vi "GetConditions.vi"(6 "condition type":T3, 7 "data group":string, 8 "error in (no error)":errorcluster, 9 "operating state":i32, 11 "operating states in":variant) -> (0 "error out":errorcluster, 1 "expression":string, 2 "conditions":T1[](array[typedef]), 3 "operating states out":variant, 4 "weight":i32)   [LabVIEW 2017, in "OpState.lvlib"]
uses:
  <vilib>/addons/InsightCM/Devices/Shared/Common/OpState/OpState.lvlib
  <vilib>/addons/InsightCM/Devices/Shared/Common/OpState/controls/ConditionType.ctl
  <vilib>/addons/InsightCM/Devices/Shared/Common/Trigger/controls/TriggerCondition.ctl
  <vilib>/addons/InsightCM/MessageBus/Base/controls/Condition.ctl
  <vilib>/addons/InsightCM/Devices/Shared/Common/OpState/controls/TriggerOperatingState.ctl
  <vilib>/addons/InsightCM/MessageBus/Base/controls/KeyValuePair.ctl
  <vilib>/addons/InsightCM/Devices/Shared/Common/Trigger/Trigger.lvlib
  <vilib>/addons/InsightCM/Utilities/PropertyHelpers/PropertyHelpers.lvlib
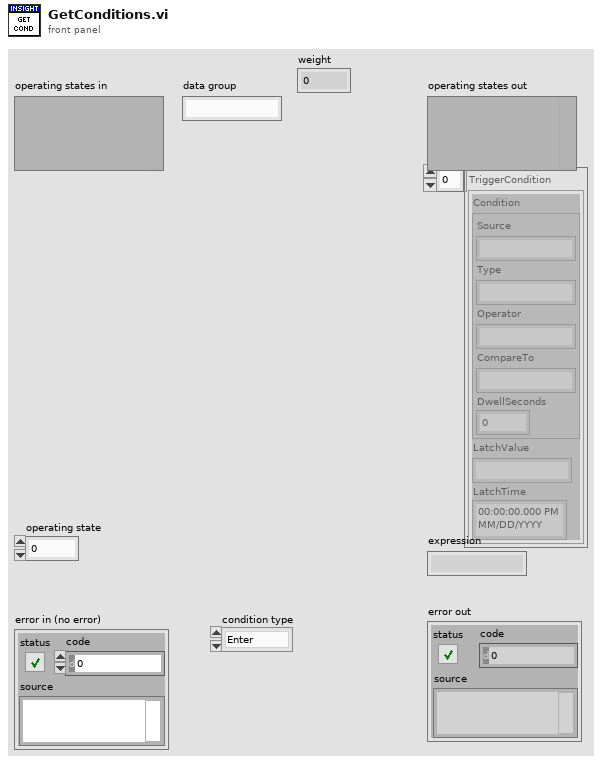
[diagram p1: front panel]
types:
  T1 = typedef "Trigger.lvlib/TriggerCondition.ctl" = cluster{"Condition":T2, "LatchValue":string, "LatchTime":timestamp}
  T2 = typedef "Condition.ctl" = cluster{"Source":string, "Type":string, "Operator":string, "CompareTo":string, "DwellSeconds":dbl}
  T3 = typedef "OpState.lvlib/ConditionType.ctl" = enum16{"Enter", "Exit"}
  T4 = typedef "OpState.lvlib/TriggerOperatingState.ctl" = cluster{"Id":string, "Name":string, "Properties":T5[], "EnterExpression":string, "EnterConditions":T1[], "ExitExpression":string, "ExitConditions":T1[]}
  T5 = typedef "KeyValuePair.ctl" = cluster{"Key":string, "Value":string}
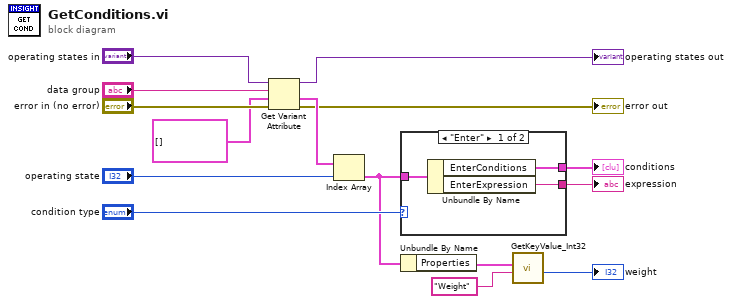
[diagram p0: block diagram]
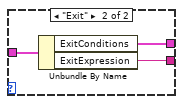
[diagram p2: hidden frame]
diagram:
  n1 = Get Variant Attribute(Variant="operating states in", name="data group", default value (empty Variant)=T4[] [] ("OperatingStates"), error in="error in (no error)") -> (duplicate Variant=→"operating states out":variant, value=w11:T4[], error out=→"error out":errorcluster)  [unwired: 1 out]
  n2 = Index Array(array=w11, index="operating state") -> (element=w4:T4)
  n3 = case shown="\"Enter\"" "condition type" {
    tunnel: w4 -> [w18 w21]
    tunnel: [w17 w20] -> w7
    tunnel: [w16 w19] -> w6
    frame "Enter" {
      n4 = Unbundle By Name(w18) -> ("EnterConditions"=w17:T1[], "EnterExpression"=w16:string)
    }
    frame "Exit" {
      n5 = Unbundle By Name(w21) -> ("ExitConditions"=w20:T1[], "ExitExpression"=w19:string)
    }
  }
  "conditions" <- w7
  "expression" <- w6
  n6 = Unbundle By Name(w4) -> ("Properties"=w3:T5[])
  n7 = call <vilib>:"GetKeyValue_Int32.vi"("key"="Weight", "key value pairs"=w3) -> ("value"=→"weight":i32)  [unwired: 7 in, 2 out]
